vi "Time.vi"() -> ()   [LabVIEW 2017, in "Examples.lvlib"]
uses:
  Examples.lvlib
panel:
  out "Logging?":bool
  in  "Start Time":timestamp
  in  "Stop Time":timestamp
  in  "Delay Time (s)":dbl=1.0
  in  "?":bool
  out "Waveform Chart":dynamicdata(graph)
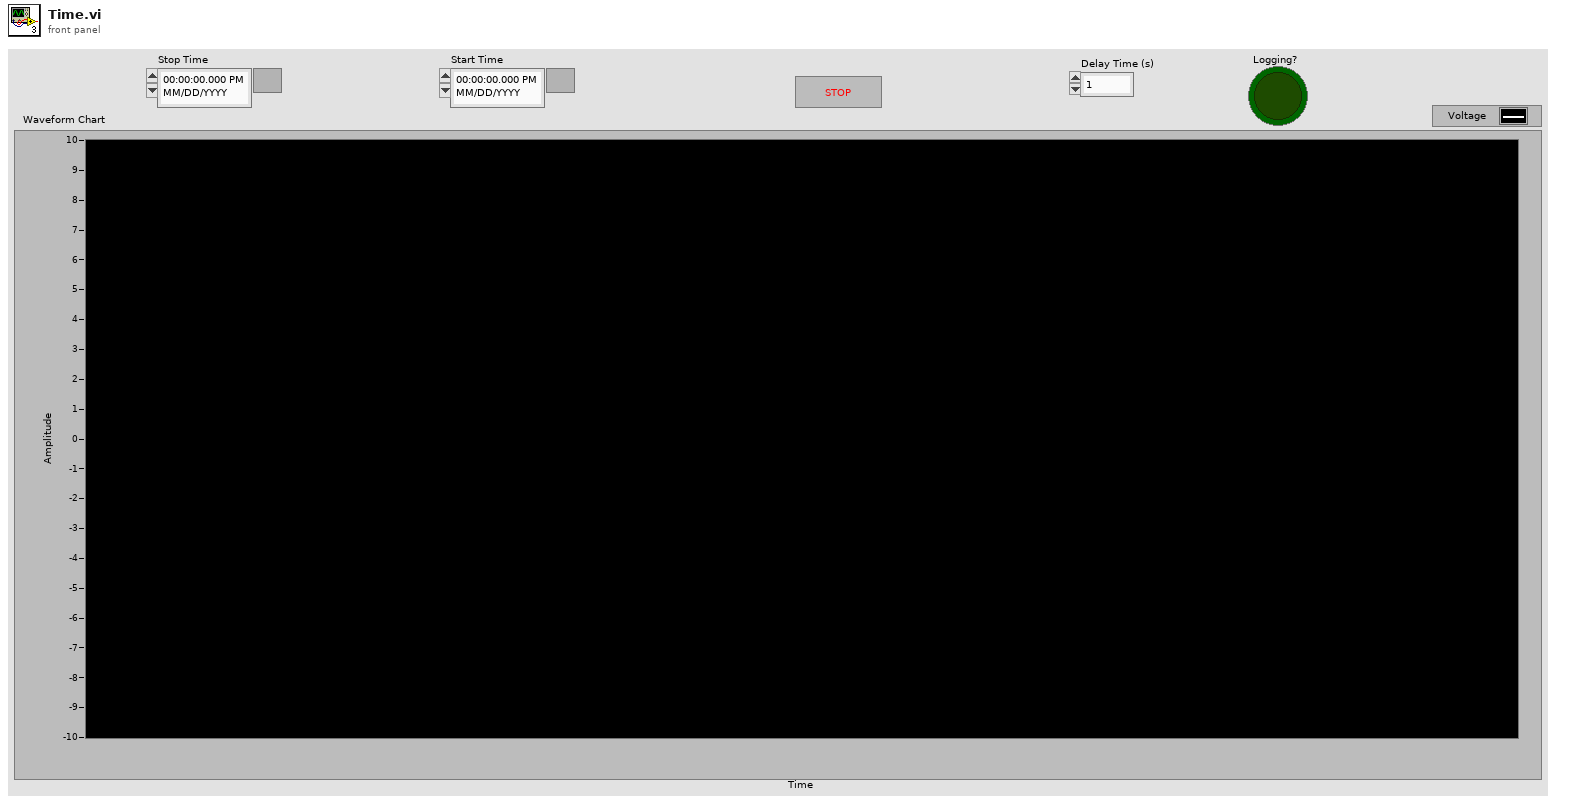
[diagram p1: front panel]
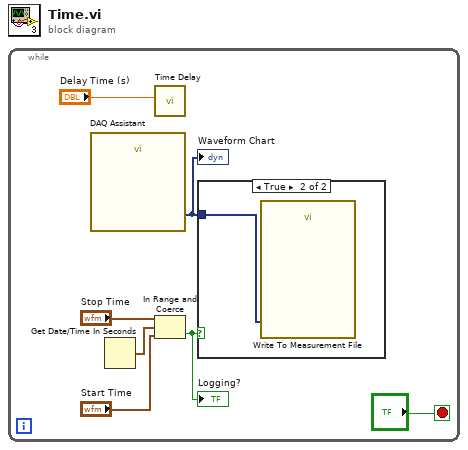
[diagram p0: block diagram]
diagram:
  n1 = while {
    stop <- "?" stop-if-true
    n2 = call "DAQ Assistant"() -> ("data"=w5:dynamicdata)  [unwired: 17 in, 2 out]
    "Waveform Chart" <- w5
    n3 = Get Date/Time In Seconds() -> (seconds since 1Jan1904=w4:timestamp)
    n4 = call "Time Delay"("Delay Time (s)"="Delay Time (s)") -> ()  [unwired: 10 in, 1 out]
    n5 = In Range and Coerce(upper limit="Stop Time", x=w4, lower limit="Start Time") -> (In Range?=w1:bool)  [unwired: 1 out]
    "Logging?" <- w1
    n6 = case shown="True" w1 {
      tunnel: w5 -> [_ w8]
      frame False {
      }
      frame True {
        n7 = call "Write To Measurement File"("Signals"=w8) -> ()  [unwired: 16 in, 3 out]
      }
    }
  }
